vi "Execute Query.vi"(7 "Timeout (15s)":i32, 8 "error in (no error)":errorcluster, 9 "Parâmetros":T1[](array[typedef]), 10 "SQL query":string, 11 "Connection in":T2) -> (0 "error out":errorcluster, 1 "Query Time":dbl, 2 "data":string[][](array[string]), 3 "Connection out":T2, 4 "Sem dados?":bool)   [LabVIEW 2020, in "Oracle Driver.lvlib"]
uses:
  Oracle Driver.lvlib
  <vilib>/addons/database/Connection.llb/Conn ObjectReference.ctl
  <vilib>/addons/database/Connection.llb/Conn Execute.vi
  <vilib>/addons/database/Recordset.llb/Rec Fetch Recordset Data (R).vi
  <vilib>/addons/database/Recordset.llb/Rec Destroy - Connection.vi
  <vilib>/addons/database/NI_Database_API.lvlib
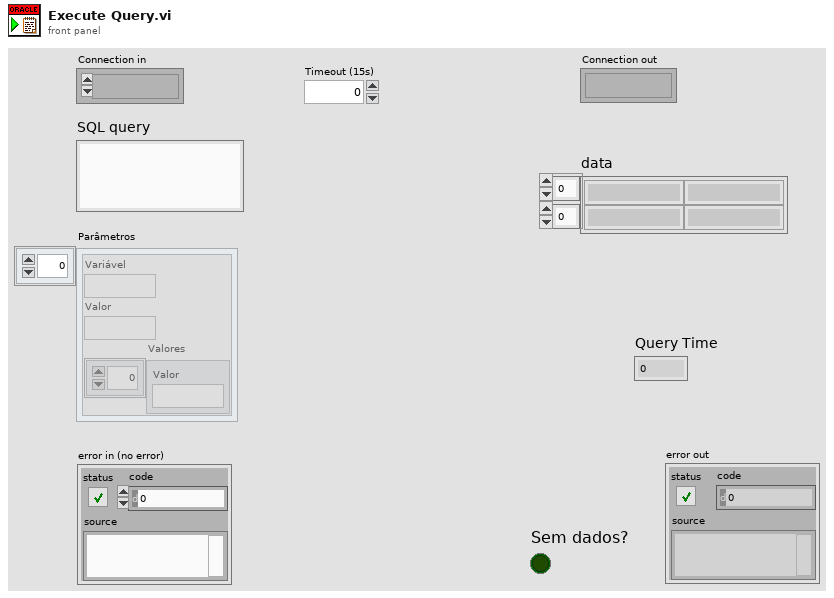
[diagram p1: front panel]
types:
  T1 = typedef "Oracle Driver.lvlib/Parâmetros.ctl" = cluster{"Variável":string, "Valor":string, "Valores":string[]}
  T2 = typedef "NI_Database_API.lvlib/Conn ObjectReference.ctl" = refnum<k1>
  T3 = typedef "NI_Database_API.lvlib/Conn DataMembers.ctl" = cluster{"ADODB._Connection":refnum<k7>, "recordset objects":i32, "command objects":i32}
  T4 = typedef "NI_Database_API.lvlib/Rec ObjectReference.ctl" = refnum<k1>
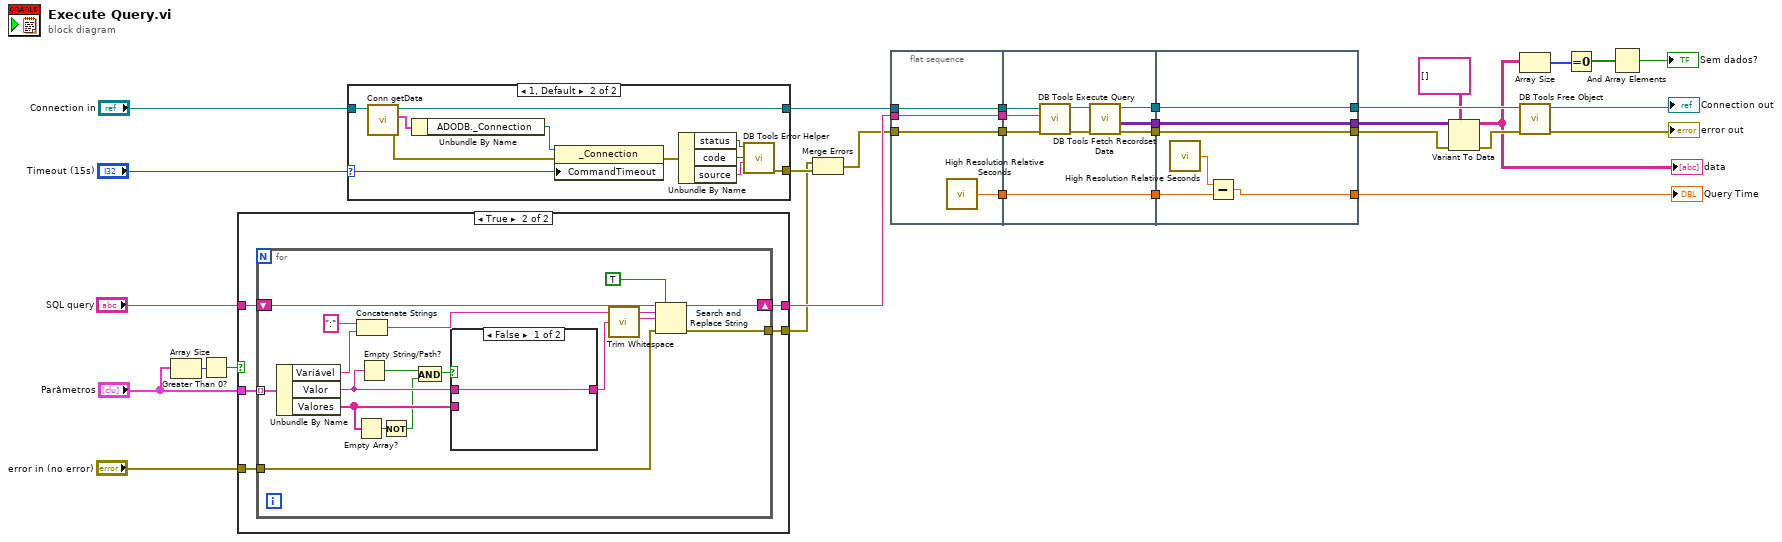
[diagram p0: block diagram]
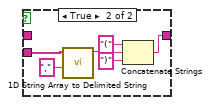
[diagram p4: hidden frame]
diagram:
  n1 = Array Size(array="Parâmetros") -> (size(s)=w16:i32)
  n2 = Greater Than 0?(x=w16) -> (x > 0?=w17:bool)
  n3 = case shown="True" w17 {
    tunnel: "Parâmetros" -> [_ w39]
    tunnel: "SQL query" -> [w34 w38]
    tunnel: [w34 w37] -> w14
    tunnel: "error in (no error)" -> [w33 w36]
    tunnel: [w33 w35] -> w1
    frame False {
    }
    frame True {
      n4 = for {
        tunnel: w39 -> [w56] mode=indexing
        shift-right: [w54] -> w37
        shift-left: w38 -> [w55]
        tunnel: w36 -> [w50]
        tunnel: [w49] -> w35
        n5 = Unbundle By Name(w56) -> ("Variável"=w52:string, "Valor"=w47:string, "Valores"=w46:string[])
        n6 = Empty Array?(array=w46) -> (empty?=w43:bool)
        n7 = Concatenate Strings(":" ("string"), w52) -> (w53:string)
        n8 = Empty String/Path?(string/path=w47) -> (empty?=w45:bool)
        n9 = Not(x=w43) -> (.not. x?=w42:bool)
        n10 = And(x=w45, y=w42) -> (x .and. y?=w44:bool)
        n11 = case shown="False" w44 {
          tunnel: w47 -> [w57 _]
          tunnel: [w57 w58] -> w41
          tunnel: w46 -> [_ w59]
          frame False {
          }
          frame True {
            n12 = call <vilib>:"1D String Array to Delimited String.vi"("delimiter"=",", "string array"=w59) -> ("delimited string"=w63:string)  [unwired: 9 in]
            n13 = Concatenate Strings("(" ("string"), w63, ")" ("string")) -> (w58:string)
          }
        }
        n14 = call <vilib>:"Trim Whitespace.vi"("string"=w41) -> ("trimmed string"=w40:string)  [unwired: 1 in]
        n15 = Search and Replace String(replace all?=TRUE ("replace all? (F)"), input string=w55, search string=w53, replace string=w40, error in=w50) -> (result string=w54:string, error out=w49:errorcluster)  [unwired: 3 in, 2 out]
      }
    }
  }
  n16 = case shown="1, Default" "Timeout (15s)" {
    selector: "Timeout (15s)" -> [_ w65]
    tunnel: "Connection in" -> [w64 w73]
    tunnel: [w64 w72] -> w5
    tunnel: [_ w66] -> w3
    frame 0 {
    }
    frame 1, Default {
      n17 = call <vilib>:"Conn getData.vi"("connection reference"=w73) -> ("error out"=w71:errorcluster, "data"=w74:T3, "connection reference out"=w72:T2)  [unwired: 1 in, 3 out]
      n18 = Unbundle By Name(w74) -> ("ADODB._Connection"=w75:refnum<k7>)
      n19 = property class="_Connection"(reference=w75, error in=w71, "CommandTimeout"=w65) -> (error out=w67:errorcluster)  [unwired: 1 out]
      n20 = Unbundle By Name(w67) -> ("status"=w69:bool, "code"=w68:i32, "source"=w70:string)
      n21 = call <vilib>:"DB Tools Error Helper.vi"("source"=w70, "code"=w68, "status"=w69) -> ("error out"=w66:errorcluster)  [unwired: 1 in, 7 out]
    }
  }
  n22 = Merge Errors(w1, w3) -> (w2:errorcluster)
  n23 = flat-sequence {
    tunnel: w14 -> [w78]
    tunnel: w5 -> [w79]
    tunnel: [w79] -> w32
    tunnel: [w78] -> w31
    tunnel: [w77] -> w30
    tunnel: w2 -> [w76]
    tunnel: [w76] -> w29
    tunnel: w32 -> [w85]
    tunnel: w31 -> [w82]
    tunnel: [w86] -> w28
    tunnel: [w84] -> w27
    tunnel: [w83] -> w26
    tunnel: w30 -> [w81]
    tunnel: [w81] -> w25
    tunnel: w29 -> [w80]
    tunnel: [w92] -> w22
    tunnel: [w93] -> w21
    tunnel: [w94] -> w19
    tunnel: w28 -> [w94]
    tunnel: w27 -> [w93]
    tunnel: w26 -> [w92]
    tunnel: w25 -> [w90]
    tunnel: [w89] -> w24
    frame #0 {
      n24 = call <vilib>:"High Resolution Relative Seconds.vi"() -> ("relative seconds"=w77:dbl)
    }
    frame #1 {
      n25 = call-poly <vilib>:"DB Tools Execute Query.vi"("error in (no error)"=w80, "SQL query"=w82, "connection reference"=w85) -> ("error out"=w88:errorcluster, "recordset reference"=w87:T4)  [unwired: 5 in]
      n26 = call-poly <vilib>:"DB Tools Fetch Recordset Data.vi"("error in (no error)"=w88, "recordset reference"=w87) -> ("error out"=w83:errorcluster, "recordset data"=w84:variant[][], "recordset reference out"=w86:T4)  [unwired: 3 in]
    }
    frame #2 {
      n27 = call <vilib>:"High Resolution Relative Seconds.vi"() -> ("relative seconds"=w91:dbl)
      n28 = Subtract(x=w91, y=w90) -> (x-y=w89:dbl)
    }
  }
  n29 = Variant To Data(error in=w22, type=string[][] [], Variant=w21) -> (data=w10:string[][], error out=w23:errorcluster)
  "data" <- w10
  n30 = Array Size(array=w10) -> (size(s)=w9:i32[])
  n31 = call-poly <vilib>:"DB Tools Free Object.vi"("error in (no error)"=w23, "recordset reference"=w19) -> ("error out"=→"error out":errorcluster, "connection reference"=→"Connection out":T2)  [unwired: 8 in]
  n32 = Equal To 0?(x=w9) -> (x = 0?=w8:bool[])
  n33 = And Array Elements(Boolean array=w8) -> (logical AND=→"Sem dados?":bool)
  "Query Time" <- w24
